vi "LV to ITX 2D AutoPlot.vi"(4 "Notes":string, 6 "X,Y,Z Labels":string[](array[string])=["x", "y"], 8 "error in":errorcluster, 9 "Z Range":T1, 10 "2D, X, Y (Cluster)":T2, 11 "path":path) -> (0 "error out":errorcluster, 3 "file":path)   [LabVIEW 2019, in "Data.ITX.lvclass"]
doc: "Write your 2D data to ITX file. This AutoPlot VI adds commands that will automatically create in Igor an intensity graph with X and Y axes scaled by the 1D arrays, allowing you to quickly view your data.\n\n-- path: base path to save data\n-- filename: base filename\n-- Notes: add any notes here to help you remember what experiment you did\n-- 2D Array: Intensity data\n-- X,Y Arrays: These are used to apply an appropriate scaling to the intensity graph\n-- X,Y wavenames: Default \"x_\" and \"y_\" are fine.\n-- X,Y,Z Labels: Labels for plotting in Igor."
uses:
  Data.ITX.lvclass
  Data/Data.lvclass
  Data/Typedefs/Operation--enum.ctl
panel:
  # "Below are relevant for creating graphs in Igor"
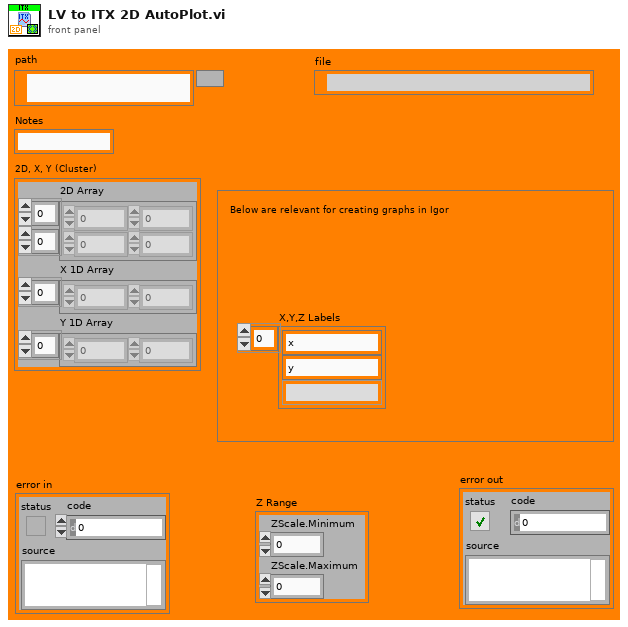
[diagram p1: front panel]
types:
  T1 = cluster{"ZScale.Minimum":dbl, "ZScale.Maximum":dbl}
  T2 = cluster{"2D Array":dbl[][], "X 1D Array":dbl[], "Y 1D Array":dbl[]}
  T3 = typedef "Data.lvclass/Operation--enum.ctl" = enum16{"Read", "Write", "Write + Append"}
  T4 = cluster{"filename without extension":string, "X wavename":string, "X  Array name":string}
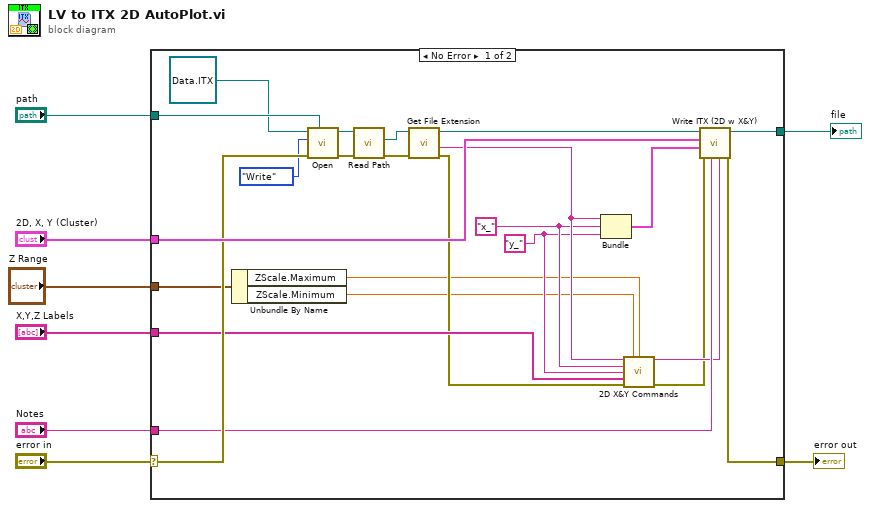
[diagram p0: block diagram]
diagram:
  n1 = case shown="No Error" "error in" {
    selector: "error in" -> [w24 w34]
    tunnel: "path" -> [w25 w33]
    tunnel: "Notes" -> [w19 _]
    tunnel: "X,Y,Z Labels" -> [w15 _]
    tunnel: [w32 w34] -> w5
    tunnel: [w31 w33] -> w4
    tunnel: "2D, X, Y (Cluster)" -> [w30 _]
    tunnel: "Z Range" -> [w11 _]
    frame No Error {
      w17 = "x_" ("X wavename")
      w16 = "y_" ("X  Array name")
      n2 = Unbundle By Name(w11) -> ("ZScale.Maximum"=w9:dbl, "ZScale.Minimum"=w10:dbl)
      n3 = call-dynamic "Open.vi"("Path"=w25, "error in (no error)"=w24, "Operation"=Operation--enum."Write", "Data in"=refnum<class "Data.ITX.lvclass"> refnum ("Data.ITX.lvclass")) -> ("error out"=w23:errorcluster, "Data out"=w22:refnum<class "Data.ITX.lvclass">)  [unwired: 6 in]
      n4 = call "Read Path.vi"("error in (no error)"=w23, "Data Save"=w22) -> ("error out"=w28:errorcluster, "Path"=w27:path)  [unwired: 7 in, 1 out]
      n5 = call <vilib>:"Get File Extension.vi"("error in (no error)"=w28, "file"=w27) -> ("error out"=w13:errorcluster, "filename without extension"=w18:string, "dup file"=w26:path)  [unwired: 5 in, 2 out]
      n6 = Bundle("filename without extension"=w18, "X wavename"=w17, "X  Array name"=w16) -> (w29:T4)  [unwired: 1 in]
      n7 = call "2D X&Y Commands.vi"("2D wave"=w18, "minimum"=w10, "maximum"=w9, "X wave"=w17, "Y wave"=w16, "X,Y,Z Labels"=w15, "error in (no error)"=w13) -> ("result string"=w14:string, "error out"=w12:errorcluster)  [unwired: 7 in]
      n8 = call "Write ITX (2D w X&Y).vi"("Commands"=w14, "Notes"=w19, "error in"=w12, "Wavenames"=w29, "2D, X, Y (Cluster)"=w30, "filename"=w26) -> ("error out"=w32:errorcluster, "file out"=w31:path)  [unwired: 3 in, 1 out]
    }
    frame Error {
    }
  }
  "file" <- w4
  "error out" <- w5
